vi "Dequeue Element String.vi"(8 "error in (no error)":errorcluster, 9 "timeout in ms (-1)":i32=-1, 11 "Priority Queue":refnum<class "Priority Queue.lvclass">) -> (0 "error out":errorcluster, 1 "timed out?":bool, 2 "Data":string, 3 "Priority Queue":refnum<class "Priority Queue.lvclass">, 4 "High Priority?":bool)   [LabVIEW 2014, in "Communicable State Machine.lvlib" / "Priority Queue.lvclass"]
uses:
  Priority Queue.lvclass
  Priority Queue.lvclass/Priority Queue.ctl
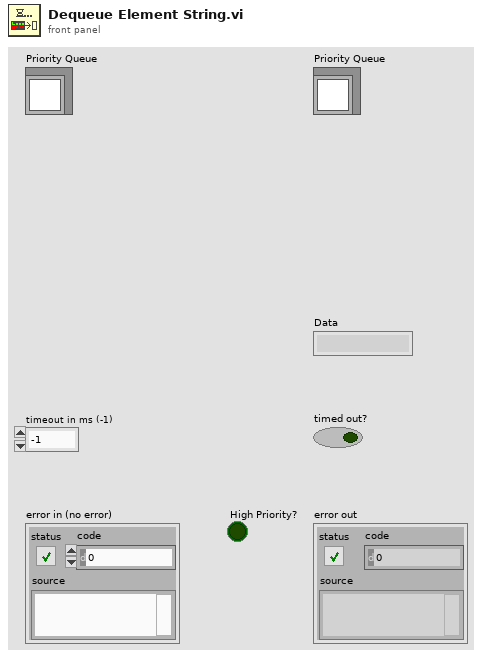
[diagram p1: front panel]
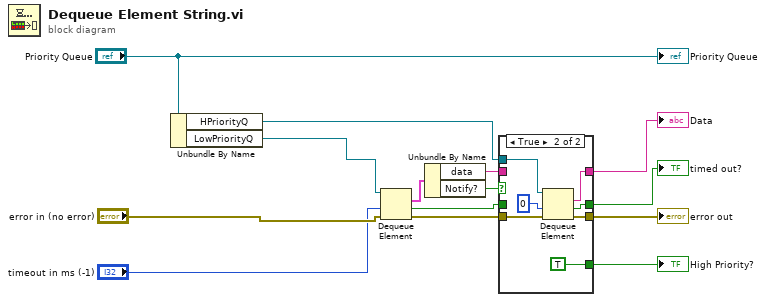
[diagram p0: block diagram]
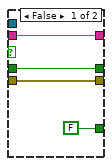
[diagram p2: hidden frame]
diagram:
  n1 = Unbundle By Name("Priority Queue") -> ("HPriorityQ"=w12:refnum<queue>, "LowPriorityQ"=w13:refnum<queue>)
  n2 = Dequeue Element(queue=w13, timeout in ms (-1)="timeout in ms (-1)", error in (no error)="error in (no error)") -> (element=w5:cluster{"data":string, "Notify?":bool}, timed out?=w2:bool, error out=w1:errorcluster)  [unwired: 1 out]
  n3 = Unbundle By Name(w5) -> ("data"=w3:string, "Notify?"=w4:bool)
  n4 = case shown="True" w4 {
    tunnel: w12 -> [_ w25]
    tunnel: w3 -> [w18 _]
    tunnel: [w18 w23] -> w8
    tunnel: [FALSE TRUE] -> w9
    tunnel: [w16 w21] -> w10
    tunnel: w2 -> [w16 _]
    tunnel: w1 -> [w15 w20]
    tunnel: [w15 w19] -> w14
    frame False {
    }
    frame True {
      n5 = Dequeue Element(queue=w25, timeout in ms (-1)=0, error in (no error)=w20) -> (element=w23:string, timed out?=w21:bool, error out=w19:errorcluster)  [unwired: 1 out]
    }
  }
  "error out" <- w14
  "timed out?" <- w10
  "High Priority?" <- w9
  "Data" <- w8
  "Priority Queue" <- "Priority Queue"
